vi "convert NI 9211 CJC to temperature.vi"(1 "CJC Channel":u32) -> (0 "CJC Temperature (C)":sgl)   [LabVIEW 2011]
doc: "This VI converts the CJC voltage read from the CJC channel on a cRIO-9211 to temperature in degrees C."
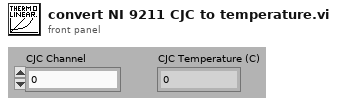
[diagram p1: front panel]
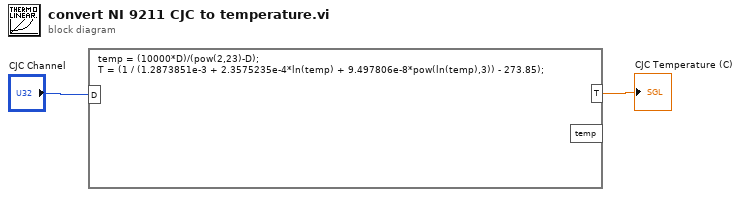
[diagram p0: block diagram]
diagram:
  n1 = formula code="temp = (10000*D)/(pow(2,23)-D);\nT = (1 / (1.2873851e-3 + 2.3575235e-4*ln(temp) + 9.497806e-8*pow(ln(temp),3)) - 273.85);"("D"="CJC Channel") -> ("T"=→"CJC Temperature (C)":dbl)  [unwired: 1 out]
